vi "Read Case ID.vi"(8 "error in (no error)":errorcluster, 11 "Consumer Msg in":refnum<class "Consumer Msg.lvclass">) -> (0 "error out":errorcluster, 2 "Case ID":string, 3 "Consumer Msg out":refnum<class "Consumer Msg.lvclass">)   [LabVIEW 2026, in "TALOS.lvlib" / "Father of all uServices.lvlib" / "Consumer Msg.lvclass"]
uses:
  Consumer Msg.lvclass
  Consumer Msg.lvclass/Consumer Msg.ctl
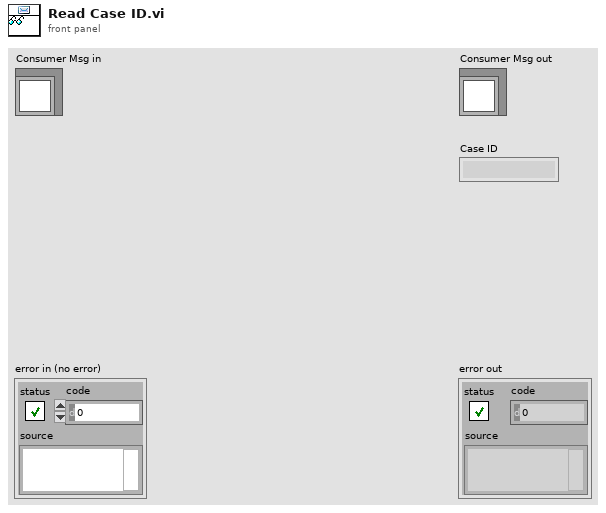
[diagram p1: front panel]
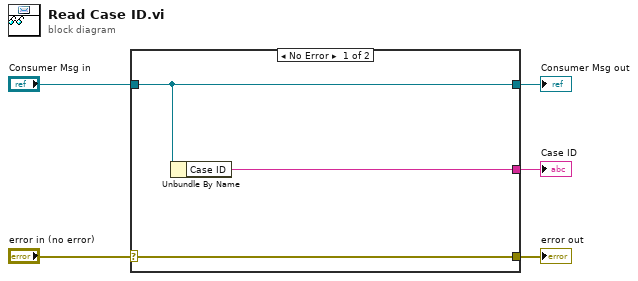
[diagram p0: block diagram]
diagram:
  n1 = case shown="No Error" "error in (no error)" {
    selector: "error in (no error)" -> [w8 w9]
    tunnel: [w8 w9] -> w4
    tunnel: [w7 w10] -> w2
    tunnel: "Consumer Msg in" -> [w7 w10]
    tunnel: [w6 _] -> w1
    frame No Error {
      n2 = Unbundle By Name(w7) -> ("Case ID"=w6:string)
    }
    frame Error {
    }
  }
  "error out" <- w4
  "Consumer Msg out" <- w2
  "Case ID" <- w1
